vi "Set He Line.vi"(8 "error in (no error)":errorcluster, 9 "Interlock Chain":refnum<class "Interlock Chain.lvclass">, 10 "Open/Close (Close)":bool, 11 "He Line in":refnum<class "He Line.lvclass">) -> (0 "error out":errorcluster, 3 "He Line out":refnum<class "He Line.lvclass">)   [LabVIEW 2015, in "cRIO-Carbondioxide.lvlib" / "CO2-Actor.lvlib" / "He Line.lvclass"]
uses:
  He Line.lvclass
  Interlocks/Interlock Chain/Interlock Chain.lvclass
  Valve/Valve.lvclass
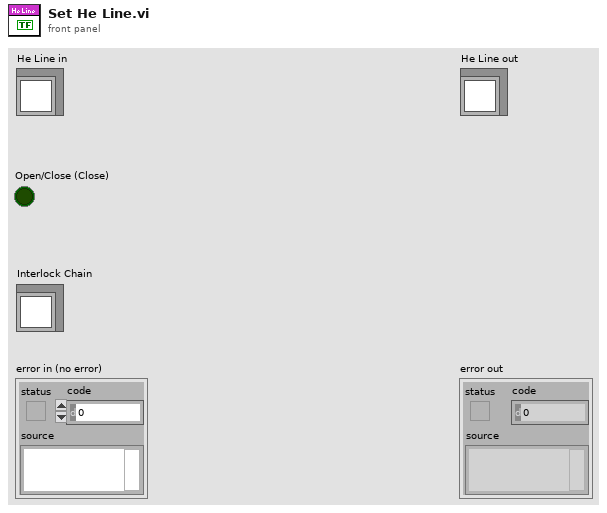
[diagram p1: front panel]
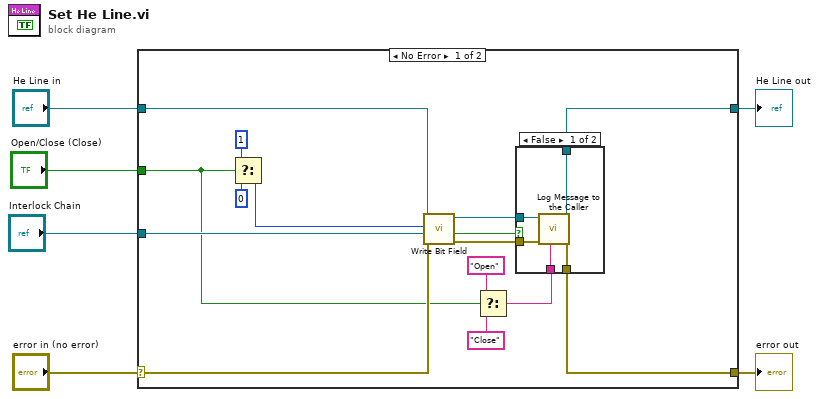
[diagram p0: block diagram]
diagram:
  n1 = case shown="No Error" "error in (no error)" {
    selector: "error in (no error)" -> [w20 w30]
    tunnel: [w11 w30] -> w5
    tunnel: [w14 w29] -> w3
    tunnel: "He Line in" -> [w21 w29]
    tunnel: "Interlock Chain" -> [w19 _]
    tunnel: "Open/Close (Close)" -> [w13 _]
    frame No Error {
      n2 = Select(t=u16 1, s=w13, f=u16 0 ("Bit Field")) -> (s? t:f=w16:u16)
      n3 = call "Write Bit Field.vi"("error in (no error)"=w20, "Interlock Chain"=w19, "Bit Field"=w16, "Valve in"=w21) -> ("error out"=w12:errorcluster, "Interlock occured?"=w7:bool, "Valve out"=w15:refnum<class "He Line.lvclass">)  [unwired: 5 in]
      n4 = Select(t="Open", s=w13, f="Close") -> (s? t:f=w10:string)
      n5 = case shown="False" w7 {
        tunnel: w15 -> [w26 w28]
        tunnel: [w25 w28] -> w14
        tunnel: w12 -> [w24 w27]
        tunnel: [w23 w27] -> w11
        tunnel: w10 -> [w22 _]
        frame False {
          n6 = call-dynamic "Log Message to the Caller.vi"("String (\"\" = no message to send)"=w22, "error in (no error)"=w24, "CO2 Actor in"=w26) -> ("error out"=w23:errorcluster, "CO2 Actor out"=w25:refnum<class "He Line.lvclass">)  [unwired: 7 in]
        }
        frame True {
        }
      }
    }
    frame Error {
    }
  }
  "error out" <- w5
  "He Line out" <- w3
